vi "_Read.vi"(8 "error in (no error)":errorcluster, 10 "Count":i32, 11 "TCP Stream in":refnum<class "TCP Stream.lvclass">) -> (0 "error out":errorcluster, 2 "Data":string, 3 "TCP Stream out":refnum<class "TCP Stream.lvclass">)   [LabVIEW 2020, in "Stream-TCP.lvlib" / "TCP Stream.lvclass"]
uses:
  TCP Stream.lvclass
  C:/Program Files (x86)/National Instruments/LabVIEW 2020/vi.lib/IlluminatedG/lv-stream/stream/Stream.lvclass
  TCP Stream.lvclass/TCP Stream.ctl
  <vilib>/IlluminatedG/lv-stream/stream/Stream.lvclass
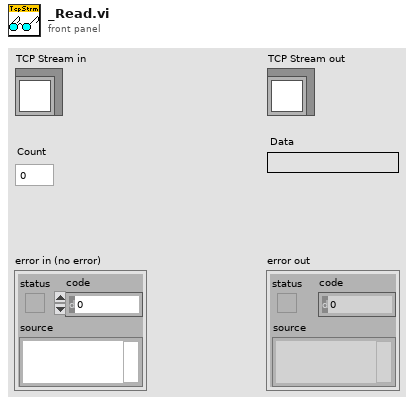
[diagram p1: front panel]
types:
  T1 = typedef "Stream.lvlib/Mode.ctl" = enum16{"Raw", "Buffered", "LineTerm"}
  T2 = enum16{"Standard", "Buffered", "CRLF", "Immediate"}
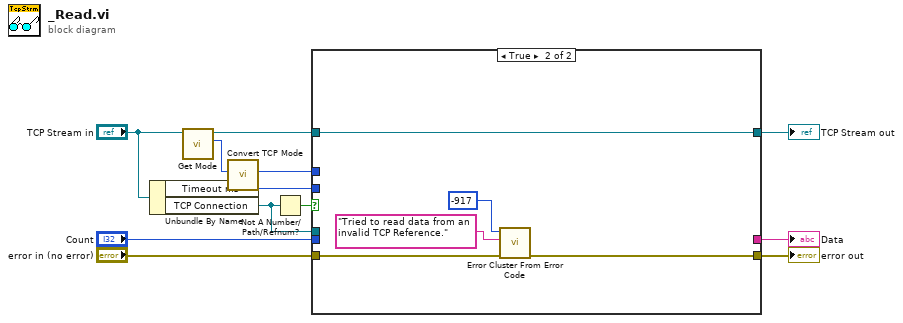
[diagram p0: block diagram]
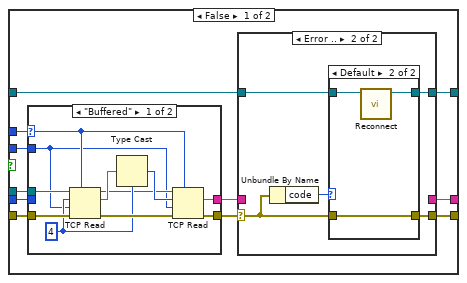
[diagram p2: hidden frame]
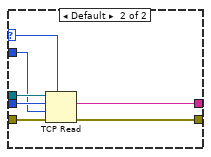
[diagram p5: hidden frame]
diagram:
  n1 = Unbundle By Name("TCP Stream in") -> ("Timeout ms"=w10:i32, "TCP Connection"=w6:refnum<k5>)
  n2 = call <vilib>:"Get Mode.vi"("Stream in"="TCP Stream in") -> ("Mode"=w2:T1, "Stream out"=w1:refnum<class "TCP Stream.lvclass">)  [unwired: 8 in, 1 out]
  n3 = call "Convert TCP Mode.vi"("Mode"=w2) -> ("TCP Mode"=w3:T2)  [unwired: 10 in]
  n4 = Not A Number/Path/Refnum?(number/path/refnum=w6) -> (NaN/Path/Refnum?=w5:bool)
  n5 = case shown="True" w5 {
    tunnel: "Count" -> [w23 _]
    tunnel: w1 -> [w21 w59]
    tunnel: [w20 w59] -> w11
    tunnel: w3 -> [w19 _]
    tunnel: w10 -> [w18 _]
    tunnel: [w16 _] -> w9
    tunnel: "error in (no error)" -> [w15 w56]
    tunnel: [w14 w55] -> w7
    tunnel: w6 -> [w13 _]
    frame False {
      n6 = case shown="\"Buffered\"" w19 {
        selector: w19 -> [w40 w48]
        tunnel: w13 -> [w46 w54]
        tunnel: w15 -> [w45 w53]
        tunnel: w23 -> [_ w52]
        tunnel: [w38 w51] -> w22
        tunnel: [w39 w50] -> w17
        tunnel: w18 -> [w37 w49]
        frame "Buffered" {
          w43 = 4
          n7 = TCP Read(connection ID=w46, bytes to read=w43, error in (no error)=w45, 7:w40, 9:w37) -> (connection ID out=w41:refnum<k5>, data out=w44:string, error out=w47:errorcluster)
          n8 = Type Cast(type=w43, x=w44) -> (*(type *) &x=w42:i32)
          n9 = TCP Read(connection ID=w41, bytes to read=w42, error in (no error)=w47, 7:w40, 9:w37) -> (data out=w39:string, error out=w38:errorcluster)  [unwired: 1 out]
        }
        frame Default {
          n10 = TCP Read(connection ID=w54, bytes to read=w52, error in (no error)=w53, 7:w48, 9:w49) -> (data out=w50:string, error out=w51:errorcluster)  [unwired: 1 out]
        }
      }
      n11 = case shown="Error .." w22 {
        selector: w22 -> [w24 w31]
        tunnel: [w24 w30] -> w14
        tunnel: w21 -> [w26 w29]
        tunnel: [w26 w28] -> w20
        tunnel: w17 -> [w25 _]
        tunnel: [w25 _] -> w16
        frame No Error {
        }
        frame Error {
          n12 = Unbundle By Name(w31) -> ("code"=w27:i32)
          n13 = case shown="Default" w27 {
            tunnel: w29 -> [w33 w36]
            tunnel: [w33 w35] -> w28
            tunnel: w31 -> [w32 w34]
            tunnel: [w32 w34] -> w30
            frame 56 {
            }
            frame Default {
              n14 = call "Reconnect.vi"("TCP Stream in"=w36) -> ("TCP Stream out"=w35:refnum<class "TCP Stream.lvclass">)  [unwired: 9 in, 1 out]
            }
          }
        }
      }
    }
    frame True {
      n15 = call <vilib>:"Error Cluster From Error Code.vi"("error in (no error)"=w56, "error message (\"\")"="Tried to read data from an invalid TCP Reference." ("error message (\"\")"), "error code (0)"=-917) -> ("error out"=w55:errorcluster)  [unwired: 6 in]
    }
  }
  "error out" <- w7
  "TCP Stream out" <- w11
  "Data" <- w9
